vi "SchedViewOnly.vi"(9 "schedname":string, 10 "schednum":string, 11 "SchedArray":string[][](array[string])) -> ()   [LabVIEW 2023]
uses:
  Schedule.ctl
panel:
  out "sched":string
  in  "CLose":bool
  in  "SCHEDULE":T1 caption="Multicolumn Listbox"
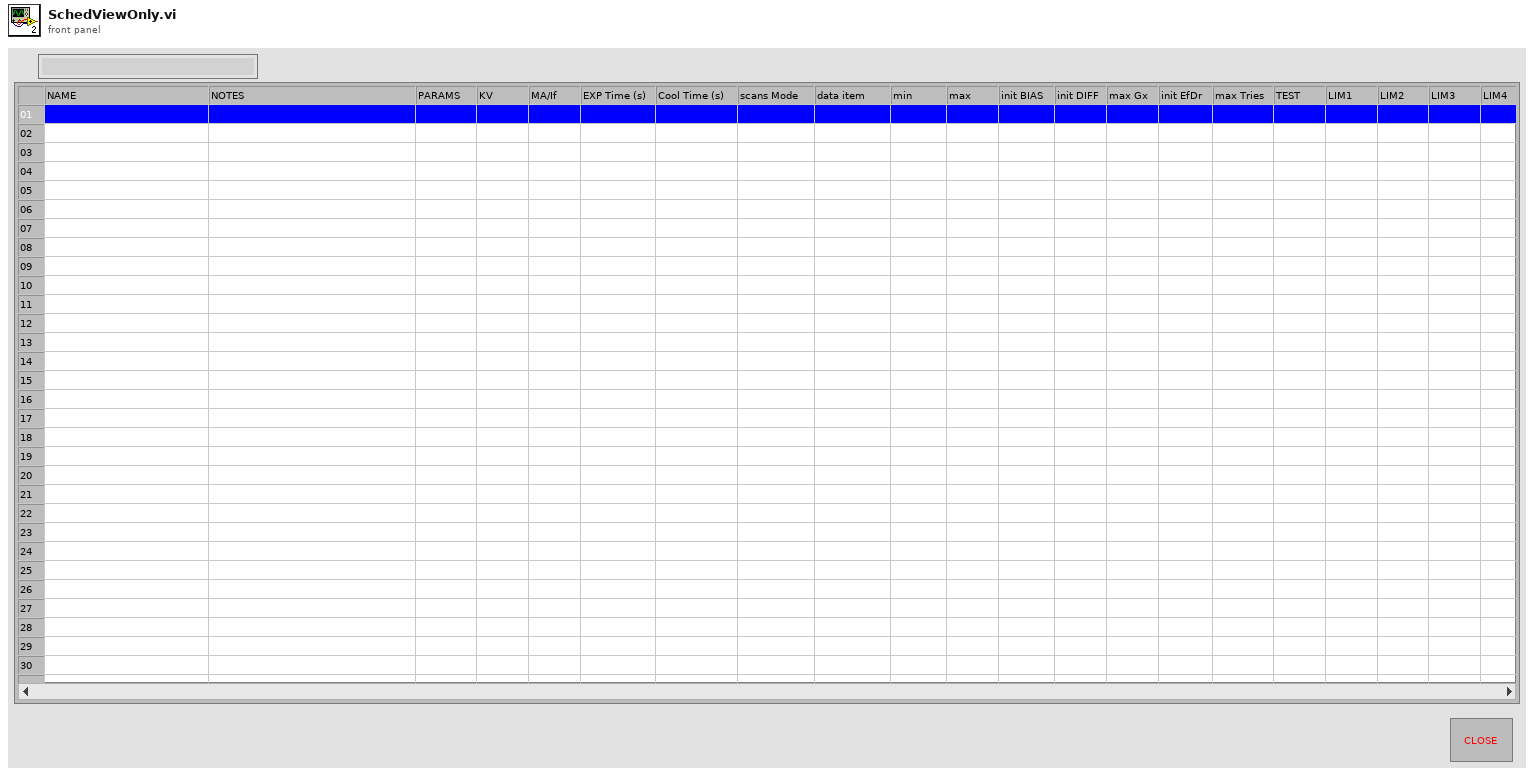
[diagram p1: front panel]
types:
  T1 = typedef "Schedule.ctl" = i32
  T2 = enum8{"Enabled", "Disabled", "Disabled and Grayed Out"}
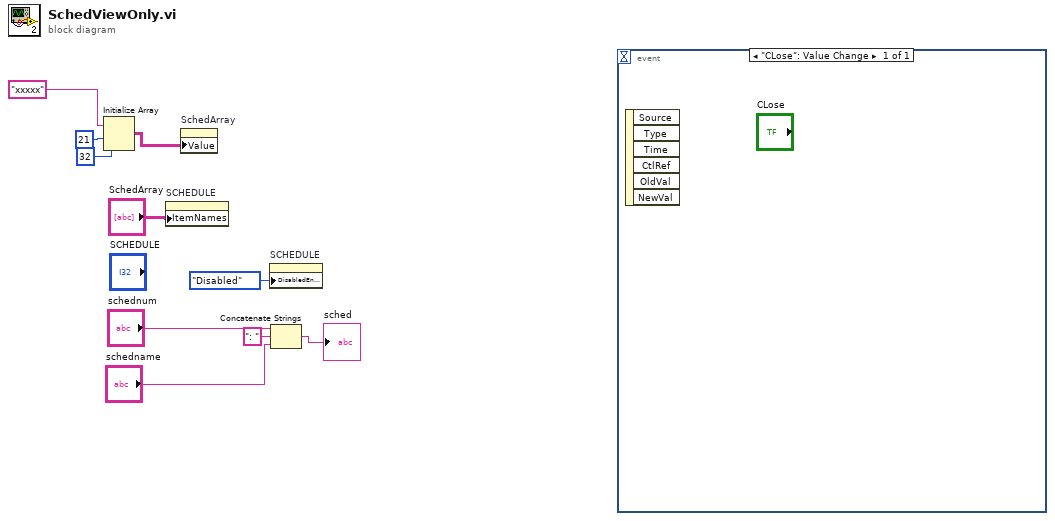
[diagram p0: block diagram]
diagram:
  n1 = Initialize Array("xxxxx", 21 ("dimension size"), 32 ("dimension size")) -> (w4:string[][])
  n2 = property on="SCHEDULE" class="MCListbox (strict)"("ItemNames"="SchedArray") -> ()  [unwired: 2 in, 2 out]
  n3 = property on="SchedArray" class="Arr (strict)"("Value"=w4) -> ()  [unwired: 2 in, 2 out]
  n4 = property on="SCHEDULE" class="MCListbox (strict)"("DisabledEnum"=T2."Disabled" ("Disabled")) -> ()  [unwired: 2 in, 2 out]
  n5 = Concatenate Strings("schednum", ": " ("string"), "schedname") -> (→"sched":string)
  n6 = event shown="[0] \"CLose\": Value Change" {
    selector: _ -> [_]
    dyn-events: _ -> [_]
    timeout: _ -> [_]
    event "CLose": Value Change {
      n7 = event-data() -> ()  [unwired: 1 in, 6 out]
    }
  }
